vi "Task Setpoint Updated.vi"(7 "Task Ident":string, 8 "error in":errorcluster, 9 "Data":variant, 10 "Setpoint Ident":string, 11 "ISeries Actor in":refnum<class "ISeries Actor.lvclass">) -> (0 "error out":errorcluster, 3 "ISeries Actor out":refnum<class "ISeries Actor.lvclass">)   [LabVIEW 2024, in "ISeries Actor.lvlib" / "ISeries Actor.lvclass"]
uses:
  ISeries Actor.lvclass
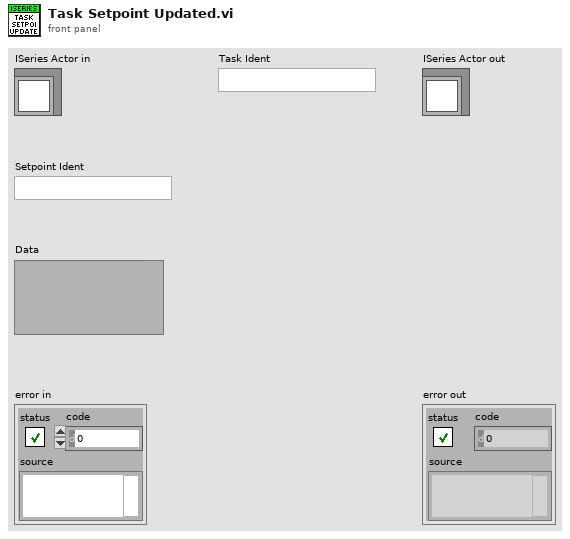
[diagram p1: front panel]
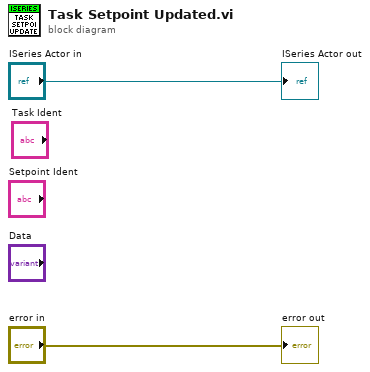
[diagram p0: block diagram]
diagram:
  "error out" <- "error in"
  "ISeries Actor out" <- "ISeries Actor in"
